vi "GetArrayXMLElement.vi"(8 "error in (no error)":errorcluster, 10 "XPathExpression":string, 11 "XMLString":string) -> (0 "error out":errorcluster, 1 "DataStringArrar":string[](array[string]), 2 "XMLStringArray":string[](array[string]))   [LabVIEW 2014, in "Project.lvclass"]
uses:
  Project.lvclass
  <vilib>/xml/Load XML String.vi
  <vilib>/xml/Close Reference(Node).vi
  <vilib>/xml/NI_XML.lvlib
  <resource>/objmgr/DOMUserDefRef.rc
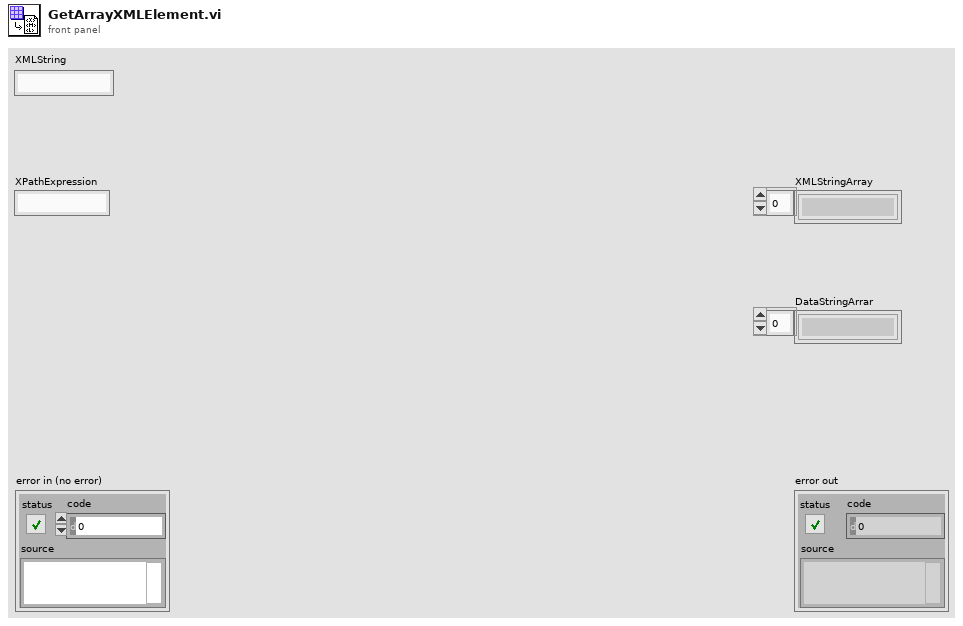
[diagram p1: front panel]
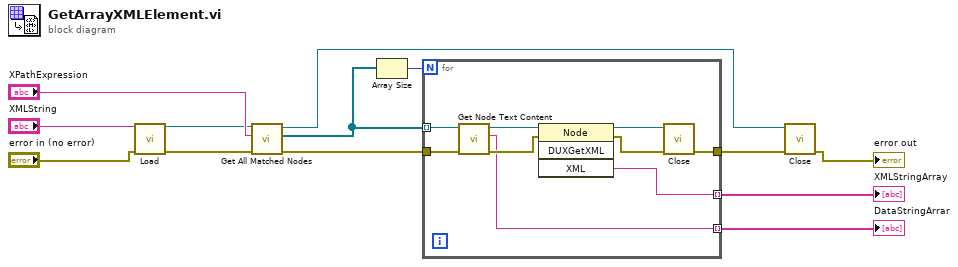
[diagram p0: block diagram]
diagram:
  n1 = call-poly <vilib>:"Load.vi"("XML string"="XMLString", "error in (no error)"="error in (no error)") -> ("DOM document out"=w9:refnum<k20>, "error out"=w8:errorcluster)  [unwired: 11 in, 1 out]
  n2 = call <vilib>:"Get All Matched Nodes.vi"("error in (no error)"=w8, "XPath expression"="XPathExpression", "node in"=w9) -> ("error out"=w13:errorcluster, "node result array"=w1:refnum<k20>[], "node out"=w6:refnum<k20>)  [unwired: 6 in]
  n3 = Array Size(array=w1) -> (size(s)=w2:i32)
  n4 = for {
    N: w2 -> [_]
    tunnel: w1 -> [w18] mode=indexing
    tunnel: w13 -> [w17]
    tunnel: [w16] -> w12
    tunnel: [w15] -> w4 mode=indexing
    tunnel: [w14] -> w3 mode=indexing
    n5 = call <vilib>:"Get Node Text Content.vi"("error in (no error)"=w17, "node in"=w18) -> ("error out"=w19:errorcluster, "node text"=w14:string, "node out"=w22:refnum<k20>)  [unwired: 7 in]
    n6 = invoke class="Node" method="DUXGetXML"(reference=w22, error in=w19) -> (reference out=w21:refnum<k20>, error out=w20:errorcluster, "XML"=w15:string)  [unwired: 2 in, 1 out]
    n7 = call-poly <vilib>:"Close.vi"("error in (no error)"=w20, "node"=w21) -> ("error out"=w16:errorcluster)  [unwired: 7 in]
  }
  "XMLStringArray" <- w4
  "DataStringArrar" <- w3
  n8 = call-poly <vilib>:"Close.vi"("error in (no error)"=w12, "node"=w6) -> ("error out"=→"error out":errorcluster)  [unwired: 7 in]
